vi "Select Page.vi"(0 "Guest Manager UI in":refnum<class "Guest Manager UI.lvclass">, 5 "Check-in":bool, 7 "Room No":string, 11 "error in (no error)":errorcluster) -> (4 "Guest Manager UI out":refnum<class "Guest Manager UI.lvclass">, 15 "error out":errorcluster)   [LabVIEW 2023, in "Guest Manager UI.lvlib" / "Guest Manager UI.lvclass"]
uses:
  Guest Manager UI.lvclass
  Guest Manager UI.lvclass/Guest Manager UI.ctl
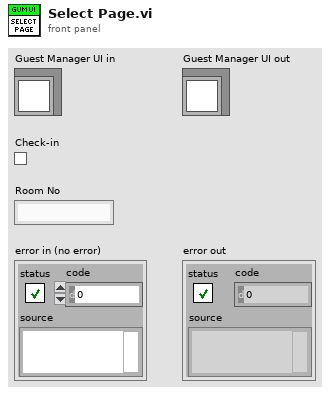
[diagram p1: front panel]
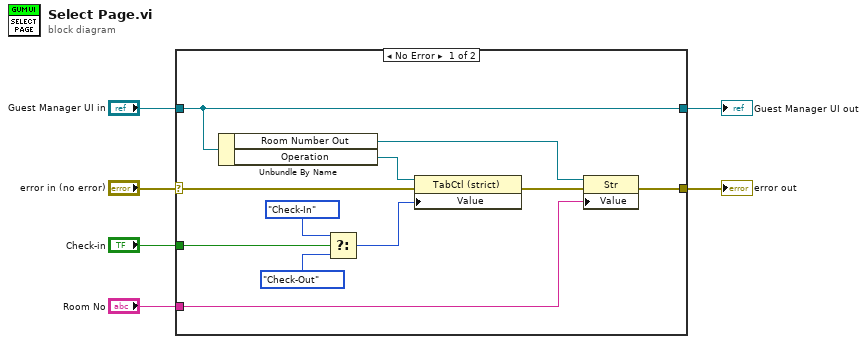
[diagram p0: block diagram]
diagram:
  n1 = case shown="No Error" "error in (no error)" {
    selector: "error in (no error)" -> [w17 w19]
    tunnel: [w9 w19] -> w5
    tunnel: [w15 w18] -> w3
    tunnel: "Guest Manager UI in" -> [w15 w18]
    tunnel: "Check-in" -> [w11 _]
    tunnel: "Room No" -> [w7 _]
    frame No Error {
      n2 = Unbundle By Name(w15) -> ("Room Number Out"=w8:refnum<vi>, "Operation"=w14:refnum<vi>)
      n3 = Select(t=enum32{"Check-In", "Check-Out"}."Check-In" ("Value"), s=w11, f=enum32{"Check-In", "Check-Out"}."Check-Out" ("Value")) -> (s? t:f=w10:enum32{"Check-In", "Check-Out"})
      n4 = property class="TabCtl (strict)"(reference=w14, error in=w17, "Value"=w10) -> (error out=w16:errorcluster)  [unwired: 1 out]
      n5 = property class="Str"(reference=w8, error in=w16, "Value"=w7) -> (error out=w9:errorcluster)  [unwired: 1 out]
    }
    frame Error {
    }
  }
  "error out" <- w5
  "Guest Manager UI out" <- w3
